vi "SL TAGS Read Server Tag.vi"(8 "error in (no error)":errorcluster, 11 "Tag Ref In":T2) -> (0 "error out":errorcluster, 3 "Tag Ref Out":T2, 5 "Aggregate Values":T1)   [LabVIEW 2017, in "EEISysLink.lvclass"]
doc: "Will input a class tag and read its value from the SystemLink server and put it in the tag variant. \n\nJames Tillett P.E.\nEndeavor Engineering Inc.\nwww.endeavoreng.com"
uses:
  EEISysLink.lvclass
  Controls/SL Tag.ctl
  <vilib>/Skyline/Tag/Wrapper/Wrapper_class/NI Skyline Tag.lvclass
  Controls/SL Tag Properties.ctl
  Controls/SL Tag Data Type.ctl
  Controls/SL Tag Interpolation Method.ctl
  Controls/SL Tag Unit of Measure.ctl
  Controls/SL Tag Type.ctl
  <vilib>/Skyline/Tag/Shared/typedefs/Tag Cluster.ctl
  <vilib>/Skyline/Tag/Shared/typedefs/DataType.ctl
  <vilib>/Skyline/Tag/Shared/typedefs/Aggregates Double.ctl
  <vilib>/Skyline/Tag/Wrapper/Wrapper_class/Read Tag (DBL).vi
  <vilib>/Skyline/Tag/Wrapper/Wrapper_class/Read Tag (String).vi
  <vilib>/Skyline/Tag/Wrapper/Wrapper_class/Read Tag (I32).vi
  <vilib>/Skyline/Tag/Shared/NI Skyline Tag.lvlib
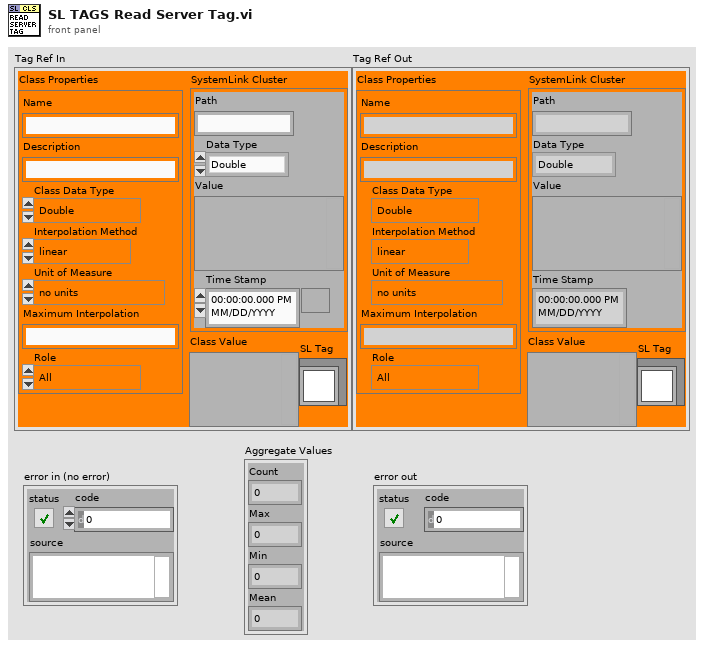
[diagram p1: front panel]
types:
  T1 = typedef "NI Skyline Tag.lvlib/Aggregates Double.ctl" = cluster{"Count":i32, "Max":dbl, "Min":dbl, "Mean":dbl}
  T2 = typedef "EEISysLink.lvclass/SL Tag.ctl" = cluster{"Class Properties":T3, "SL Tag":refnum<class "NI Skyline Tag.lvclass">, "SystemLink Cluster":T8, "Class Value":variant}
  T3 = typedef "EEISysLink.lvclass/SL Tag Properties.ctl" = cluster{"Class Data Type":T4, "Name":string, "Description":string, "Interpolation Method":T5, "Unit of Measure":T6, "Maximum Interpolation":string, "Role":T7}
  T4 = typedef "EEISysLink.lvclass/SL Tag Data Type.ctl" = enum16{"Double", "Integer", "String", "Boolean", "Waveform"}
  T5 = typedef "EEISysLink.lvclass/SL Tag Interpolation Method.ctl" = enum16{"linear", "pilinear", "step"}
  T6 = typedef "EEISysLink.lvclass/SL Tag Unit of Measure.ctl" = enum16{"no units", "Second", "Hour", "Minute", "Day", "Year", "Month", "Week", "Foot", "Yard", "Meter", "Centimeter", "Inch", "Mile", "Nautical Mile", "Miles per Hour", "Meters per second", "Square meter", "Cubic meter", "Cubic centimeter", "Cubic inch", "Liter", "Gallon", "Gallons dry US", "Gallon UK", "Percent", "Revolutions per minute", "Revolution", "Degree angle", "Astronomical Unit", "Atom", "Atomic mass", "Bar", "Byte", "C (speed of light)", "Curie", "Decibel", "Electron Volt", "Ounce", "Knot", "G", "Grade", "Are", "Hectare", "Faraday", "Franklin", "Gilbert", "Erg", "Lambert", "Maxwell", "Gauss", "Electron mass", "Kilogram force", "Pound force", "Rad", "Centiradian", "Sphere", "Mach", "Fluid Ounces", "Fluid Ounces UK", "Fahrenheit", "Celsius", "Kelvin", "Rankine", "Gram", "Kilogram", "Pound", "Short/US Ton", "Long/UK ton", "Metric ton", "Mole", "Pounds per square inch", "Inches water column", "Torr", "Millitorr", "Millimeter mercury", "Inches mercury", "Bar (2)", "Atmosphere", "Pascal", "Watt", "kiloWatt", "Horsepower", "Kilowatt Hour", "British thermal units", "Millions of BTU", "Ampere", "Candela", "Radian", "Steradian", "Bit", "Hertz", "Newton", "Joule", "Coulomb", "Volt", "Farad", "Ohm", "Siemens", "Weber", "Tesla", "Henry", "Lumen", "Lux", "Becqueral", "Gray", "Sievert", "Katal", "Angstrom", "Light Year", "Parsec", "Point", "Pixel", "Dyne", "Kilogram force (2)", "Pound force (2)", "Rem", "Rutherford", "Roentgen"}
  T7 = typedef "EEISysLink.lvclass/SL Tag Type.ctl" = enum16{"All", "Supervisor", "Worker"}
  T8 = typedef "NI Skyline Tag.lvlib/Tag Cluster.ctl" = cluster{"Path":string, "Data Type":T9, "Value":variant, "Time Stamp":timestamp}
  T9 = typedef "NI Skyline Tag.lvlib/DataType.ctl" = enum32{"Double", "Integer", "String"}
  T10 = typedef "NI Skyline Tag.lvlib/Aggregates Int.ctl" = cluster{"Count":i32, "Max":i32, "Min":i32, "Mean":dbl}
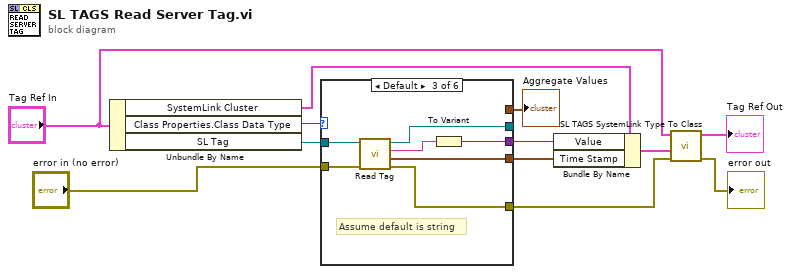
[diagram p0: block diagram]
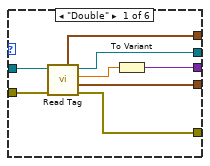
[diagram p2: hidden frame]
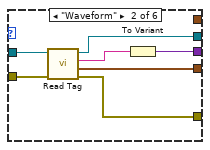
[diagram p3: hidden frame]
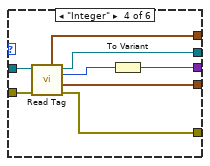
[diagram p4: hidden frame]
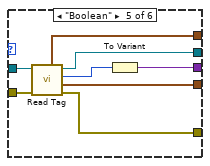
[diagram p5: hidden frame]
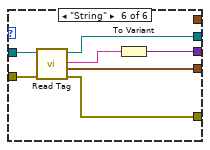
[diagram p6: hidden frame]
diagram:
  n1 = Unbundle By Name("Tag Ref In") -> ("SystemLink Cluster"=w8:T8, "Class Properties.Class Data Type"=w12:T4, "SL Tag"=w11:refnum<class "NI Skyline Tag.lvclass">)
  n2 = case shown="Default" w12 {
    tunnel: [w20 w27 w34 w42 w50 w57] -> _
    tunnel: [w19 w26 w33 w41 w49 w56] -> w6
    tunnel: "error in (no error)" -> [w17 w24 w31 w39 w47 w54]
    tunnel: w11 -> [w18 w25 w32 w40 w48 w55]
    tunnel: [w16 w23 w30 w38 w46 w53] -> w9
    tunnel: [w15 _ _ w37 w45 _] -> w2
    tunnel: [w14 w22 w29 w36 w44 w52] -> w1
    frame "Double" {
      n3 = call-poly <vilib>:"Read Tag.vi"("error in (no error)"=w17, "tag in"=w18) -> ("error out"=w19:errorcluster, "time stamp"=w16:timestamp, "value"=w13:dbl, "tag out"=w20:refnum<class "NI Skyline Tag.lvclass">, "Aggregate Values"=w15:T1)  [unwired: 5 in]
      n4 = To Variant(anything=w13) -> (Variant=w14:variant)
    }
    frame "Waveform" {
      n5 = call-poly <vilib>:"Read Tag.vi"("error in (no error)"=w24, "tag in"=w25) -> ("error out"=w26:errorcluster, "time stamp"=w23:timestamp, "value"=w21:string, "tag out"=w27:refnum<class "NI Skyline Tag.lvclass">)  [unwired: 5 in, 1 out]
      n6 = To Variant(anything=w21) -> (Variant=w22:variant)
    }
    frame Default {
      # "Assume default is string"
      n7 = call-poly <vilib>:"Read Tag.vi"("error in (no error)"=w31, "tag in"=w32) -> ("error out"=w33:errorcluster, "time stamp"=w30:timestamp, "value"=w28:string, "tag out"=w34:refnum<class "NI Skyline Tag.lvclass">)  [unwired: 5 in, 1 out]
      n8 = To Variant(anything=w28) -> (Variant=w29:variant)
    }
    frame "Integer" {
      n9 = call-poly <vilib>:"Read Tag.vi"("error in (no error)"=w39, "tag in"=w40) -> ("error out"=w41:errorcluster, "time stamp"=w38:timestamp, "value"=w35:i32, "tag out"=w42:refnum<class "NI Skyline Tag.lvclass">, "Aggregate Values"=w37:T10)  [unwired: 5 in]
      n10 = To Variant(anything=w35) -> (Variant=w36:variant)
    }
    frame "Boolean" {
      n11 = call-poly <vilib>:"Read Tag.vi"("error in (no error)"=w47, "tag in"=w48) -> ("error out"=w49:errorcluster, "time stamp"=w46:timestamp, "value"=w43:i32, "tag out"=w50:refnum<class "NI Skyline Tag.lvclass">, "Aggregate Values"=w45:T10)  [unwired: 5 in]
      n12 = To Variant(anything=w43) -> (Variant=w44:variant)
    }
    frame "String" {
      n13 = call-poly <vilib>:"Read Tag.vi"("error in (no error)"=w54, "tag in"=w55) -> ("error out"=w56:errorcluster, "time stamp"=w53:timestamp, "value"=w51:string, "tag out"=w57:refnum<class "NI Skyline Tag.lvclass">)  [unwired: 5 in, 1 out]
      n14 = To Variant(anything=w51) -> (Variant=w52:variant)
    }
  }
  "Aggregate Values" <- w2
  n15 = Bundle By Name(cluster=w8, "Value"=w1, "Time Stamp"=w9) -> (w7:T8)
  n16 = call "SL TAGS SystemLink Type To Class.vi"("error in (no error)"=w6, "SystemLink Cluster"=w7, "Class Tag In"="Tag Ref In") -> ("error out"=→"error out":errorcluster, "Class Tag Out"=→"Tag Ref Out":T2)  [unwired: 7 in]
